vi "AMC Simple Clock Example.vi"() -> ()   [LabVIEW 2017]
uses:
  <vilib>/Utility/config.llb/NI_LVConfig.lvlib
  AMC Simple Clock Style.ctl
  <vilib>/Utility/config.llb/Read Key (I32).vi
  <vilib>/Utility/config.llb/Write Key (I32).vi
panel:
  in  "Save State":bool
  out "Seconds":bool[](array[boolean])
  out "Seconds Tens":bool[](array[boolean])
  out "Minutes":bool[](array[boolean])
  out "Minutes Tens":bool[](array[boolean])
  out "Hours":bool[](array[boolean])
  out "Hours Tens":bool[](array[boolean])
  out "Digital":string
  in  "Clock Style":T1
  out "Hour":dbl(knob) scale=0.0..12.0
  out "Minute":dbl(knob) scale=0.0..12.0 scale format="%#.0f"
  out "Status":string
  in  "About":bool
  in  "Exit":bool
  in  "State Variables":cluster{"Config File":path, "Clock Style":T1}
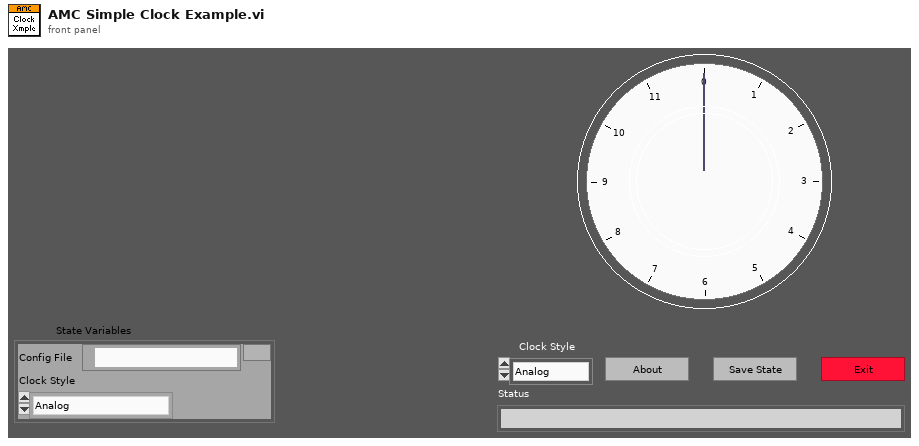
[diagram p1: front panel]
types:
  T1 = typedef "AMC Simple Clock Style.ctl" = enum16{"Analog", "Digital", "Binary"}
  T2 = typedef "amc_Message Queue.ctl" = refnum<queue>
  T3 = typedef "LVDateTimeRec.ctl" = cluster{"fractional second":dbl, "second":i32, "minute":i32, "hour":i32, "day of month":i32, "month":i32, "year":i32, "day of week":i32, "day of year":i32, "DST":i32}
  T4 = typedef "NI_LVConfig.lvlib/Config Data RefNum.ctl" = refnum<k1>
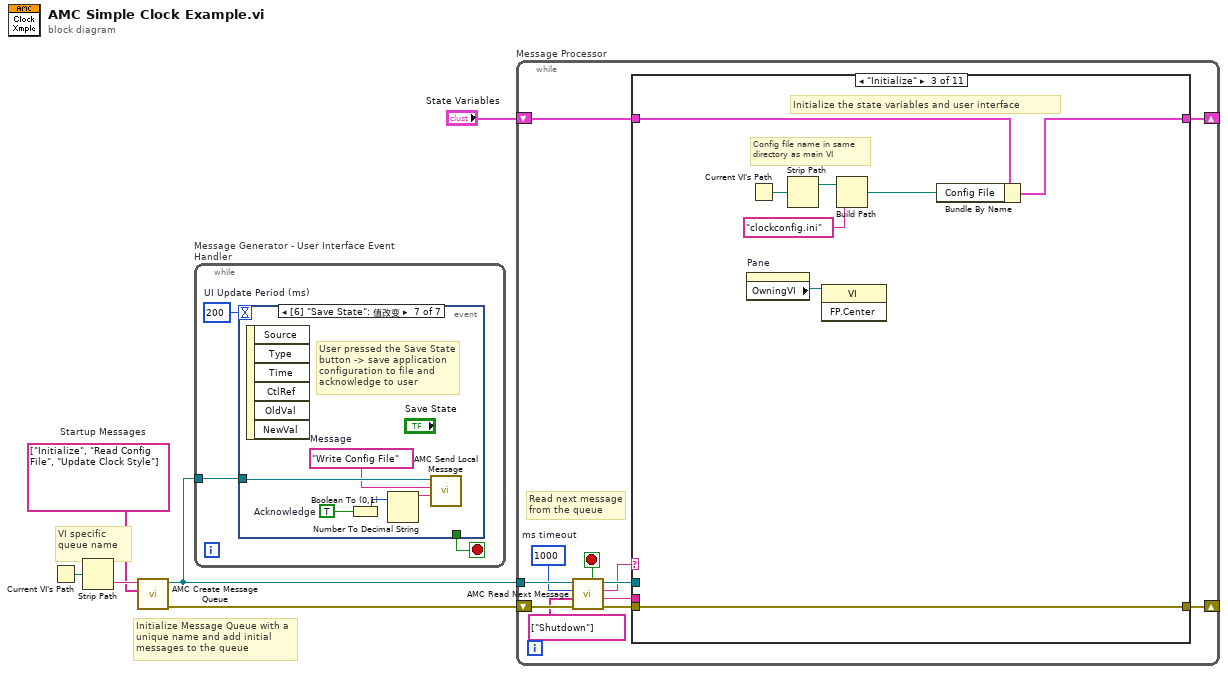
[diagram p0: block diagram]
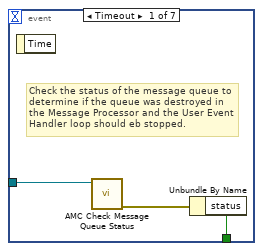
[diagram p2: hidden frame]
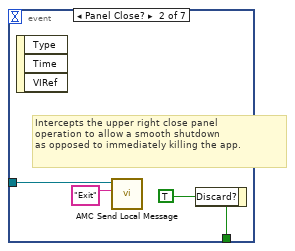
[diagram p3: hidden frame]
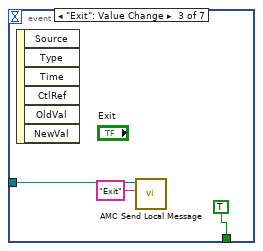
[diagram p4: hidden frame]
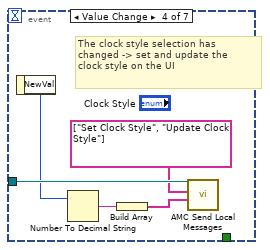
[diagram p5: hidden frame]
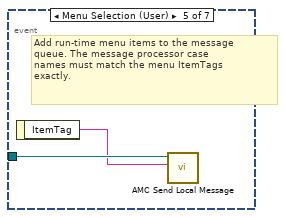
[diagram p6: hidden frame]
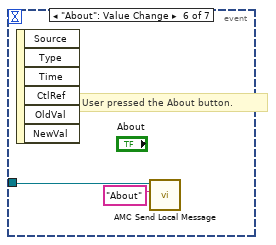
[diagram p7: hidden frame]
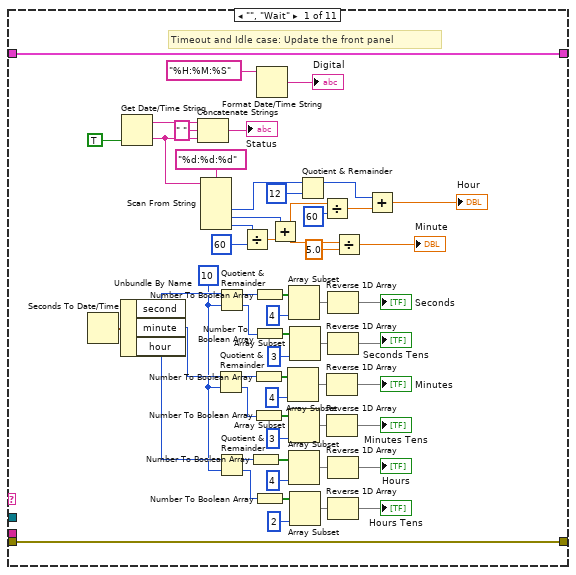
[diagram p8: hidden frame]
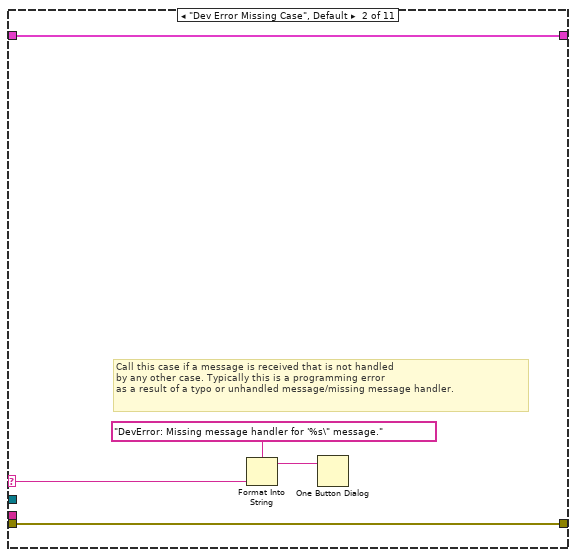
[diagram p9: hidden frame]
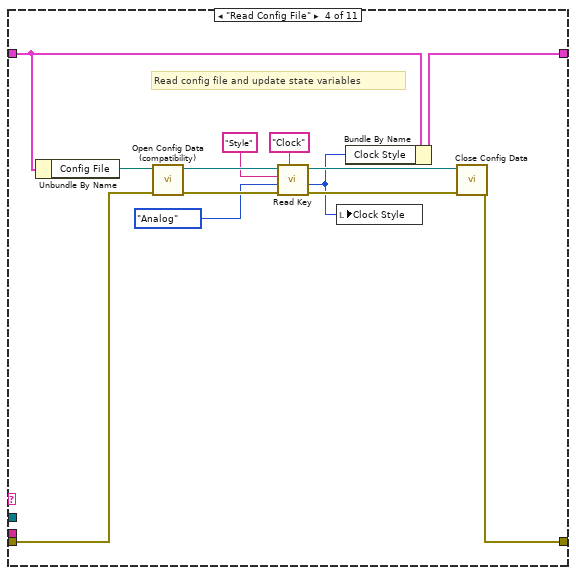
[diagram p10: hidden frame]
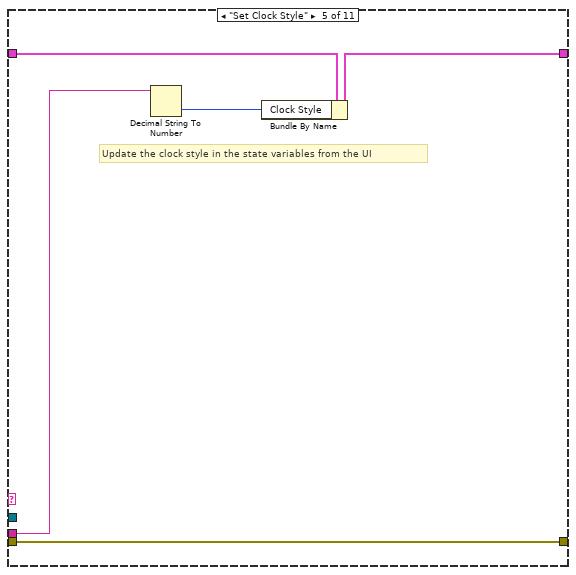
[diagram p11: hidden frame]
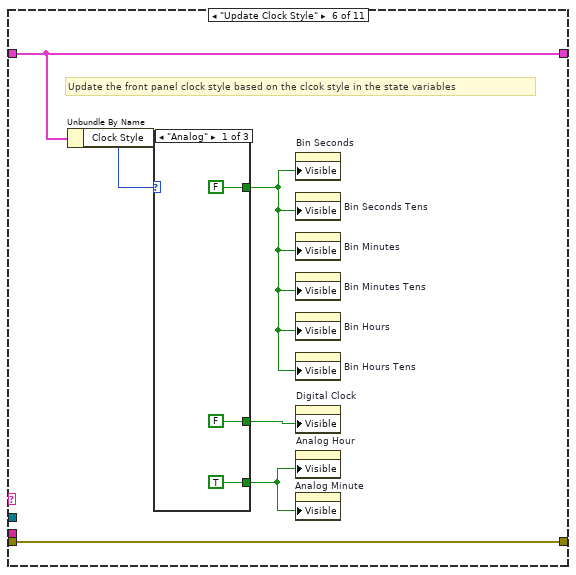
[diagram p12: hidden frame]
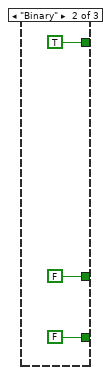
[diagram p13: hidden frame]
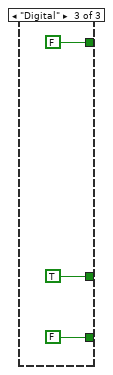
[diagram p14: hidden frame]
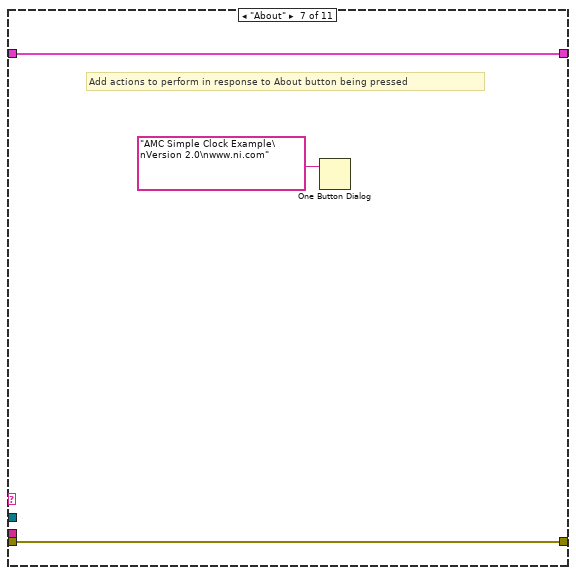
[diagram p15: hidden frame]
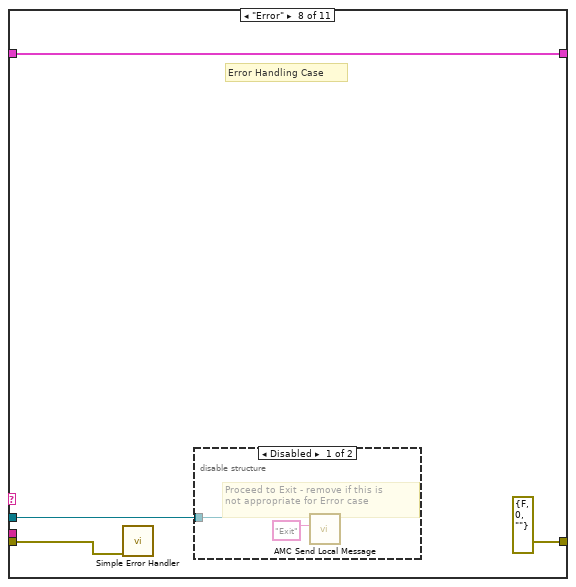
[diagram p16: hidden frame]
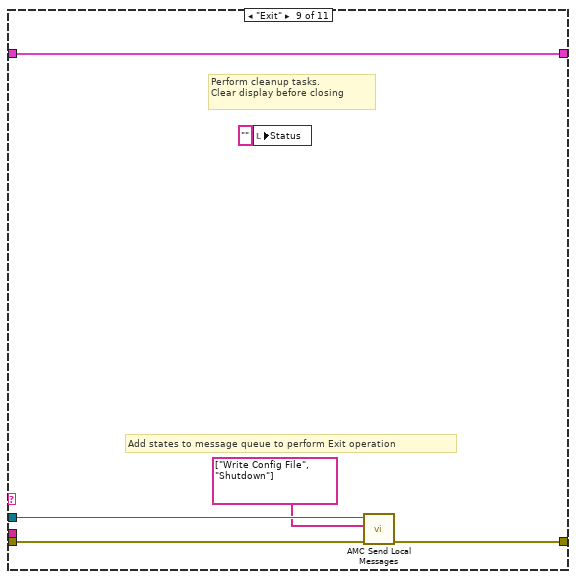
[diagram p18: hidden frame]
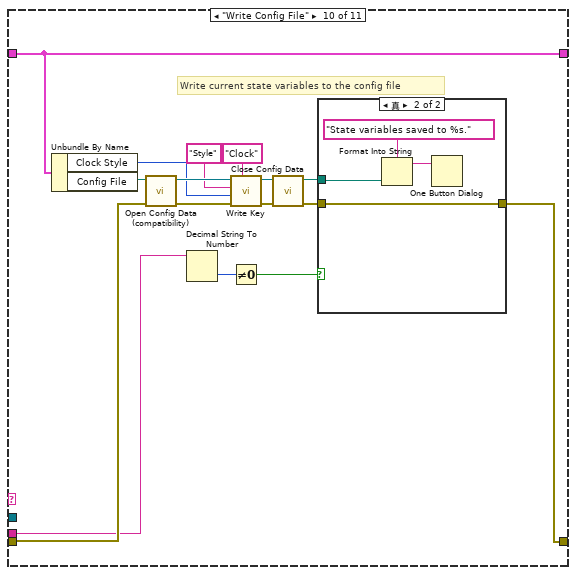
[diagram p19: hidden frame]
diagram:
  w1 = string[] ["Initialize", "Read Config File", "Update Clock Style"]  # Startup Messages
  # "VI specific\nqueue name"
  # "Initialize Message Queue with a unique name and add initial messages to the queue"
  n1 = Current VI's Path() -> (path=w3:path)
  n2 = Strip Path(path=w3) -> (name=w2:string)  [unwired: 1 out]
  n3 = call "AMC Create Message Queue.vi"("Initial Message Names"=w1, "Message Queue Name"=w2) -> ("error out"=w6:errorcluster, "Message Queue out"=w4:T2)  [unwired: 3 in, 5 out]
  n4 = while "Message Generator - User Interface Event Handler" {
    tunnel: w4 -> [w7]
    stop <- w8 stop-if-true
    w9 = 200  # UI Update Period (ms)
    n5 = event shown="[6] \"Save State\": 值改变" {
      selector: _ -> [_ _ _ _ _ _ _]
      dyn-events: _ -> [_ _ _ _ _ _ _]
      timeout: w9 -> [_ _ _ _ _ _ _]
      tunnel: [w12 w15 TRUE ("Discard?") _ _ _ _] -> w8
      tunnel: w7 -> [w11 w14 w17 w23 w25 w27 w32]
      event Timeout {
        # "Check the status of the message queue to determine if the queue was destroyed in the Message Processor and the User Event Handler loop should eb stopped."
        n6 = event-data() -> ()  [unwired: 2 out]
        n7 = call "AMC Check Message Queue Status.vi"("Message queue in"=w11) -> ("error out"=w10:errorcluster)  [unwired: 2 in, 7 out]
        n8 = Unbundle By Name(w10) -> ("status"=w12:bool)
      }
      event Panel Close? {
        w15 = TRUE ("Discard?")
        # "Intercepts the upper right close panel\noperation to allow a smooth shutdown\nas opposed to immediately killing the app."
        n9 = event-data() -> ()  [unwired: 4 out]
        n10 = call "AMC Send Local Message.vi"("Message Name"="Exit", "Message Queue in"=w14) -> ()  [unwired: 4 in, 6 out]
        n11 = event-data("Discard?"=w15) -> ()  [unwired: 1 in, 1 out]
      }
      event "Exit": Value Change {
        n12 = event-data() -> ()  [unwired: 7 out]
        n13 = call "AMC Send Local Message.vi"("Message Name"="Exit", "Message Queue in"=w17) -> ()  [unwired: 4 in, 6 out]
      }
      event Value Change {
        # "The clock style selection has\nchanged -> set and update the\nclock style on the UI"
        n14 = event-data() -> ("NewVal"=w20:T1)  [unwired: 1 out]
        n15 = Number To Decimal String(number=w20) -> (decimal integer string=w22:string)  [unwired: 1 out]
        n16 = Build Array(w22) -> (w21:string[])
        n17 = call "AMC Send Local Messages.vi"("Message Values"=w21, "Message Names"=string[] ["Set Clock Style", "Update Clock Style"], "Message Queue in"=w23) -> ()  [unwired: 2 in, 7 out]
      }
      event Menu Selection (User) {
        # "Add run-time menu items to the message\nqueue. The message processor case\nnames must match the menu ItemTags\nexactly."
        n18 = event-data() -> ("ItemTag"=w24:string)  [unwired: 1 out]
        n19 = call "AMC Send Local Message.vi"("Message Name"=w24, "Message Queue in"=w25) -> ()  [unwired: 4 in, 6 out]
      }
      event "About": Value Change {
        # "User pressed the About button."
        n20 = event-data() -> ()  [unwired: 7 out]
        n21 = call "AMC Send Local Message.vi"("Message Name"="About", "Message Queue in"=w27) -> ()  [unwired: 4 in, 6 out]
      }
      event "Save State": Value Change {
        w30 = TRUE  # Acknowledge
        w31 = "Write Config File"  # Message
        # "User pressed the Save State button -> save application configuration to file and acknowledge to user"
        n22 = event-data() -> ()  [unwired: 7 out]
        n23 = Boolean To (0,1)(Boolean=w30) -> (0, 1=w28:i16)
        n24 = Number To Decimal String(number=w28) -> (decimal integer string=w29:string)  [unwired: 1 out]
        n25 = call "AMC Send Local Message.vi"("Message Value"=w29, "Message Name"=w31, "Message Queue in"=w32) -> ()  [unwired: 3 in, 6 out]
      }
    }
  }
  n26 = while "Message Processor" {
    shift-left: w6 -> [w38]
    shift-right: [w39] -> _
    tunnel: w4 -> [w37]
    shift-left: "State Variables" -> [w44]
    shift-right: [w43] -> _
    stop <- w42 stop-if-true
    w35 = 1000  # ms timeout
    # "Read next message from the queue"
    n27 = call "AMC Read Next Message.vi"("error in (no error)"=w38, "Termination List ([Exit])"=string[] ["Shutdown"], "timeout (1ms)"=w35, "Message Queue in"=w37) -> ("error out"=w40:errorcluster, "Message Value"=w34:string, "Message Name"=w36:string, "Message Queue out"=w41:T2, "Exit Process"=w42:bool)  [unwired: 3 out]
    n28 = case shown="\"Initialize\"" w36 {
      selector: w36 -> [_ w105 _ _ _ _ _ _ _ _ _]
      tunnel: [w102 w107 w113 w124 w131 w138 w150 w155 w163 w171 w186] -> w43
      tunnel: w44 -> [w102 w107 w114 w120 w132 w138 w150 w155 w163 w171 w186]
      tunnel: w41 -> [_ _ _ _ _ _ _ w152 w161 _ w187]
      tunnel: w40 -> [w101 w106 w115 w118 w133 w139 w151 w153 w160 w170 w188]
      tunnel: [w101 w106 w115 w117 w133 w139 w151 errorcluster {"status"=FALSE, "code"=0, "source"=""} ("error out") w159 w164 w185] -> w39
      tunnel: w34 -> [_ _ _ _ w130 _ _ _ _ w169 _]
      frame "", "Wait" {
        w59 = 10 ("y")
        # "Timeout and Idle case: Update the front panel"
        n29 = Seconds To Date/Time() -> (date time rec=w85:T3)  [unwired: 2 out]
        n30 = Unbundle By Name(w85) -> ("second"=w84:i32, "minute"=w61:i32, "hour"=w60:i32)
        n31 = Get Date/Time String(want seconds? (F)=TRUE) -> (date string=w100:string, time string=w50:string)  [unwired: 2 out]
        n32 = Concatenate Strings(w100, " " ("string"), w50) -> (→"Status":string)
        n33 = Scan From String(format string="%d:%d:%d", input string=w50) -> (output 1=w46:i32, output 2=w93:i32, output 3=w86:i32)  [unwired: 2 in, 6 out]
        n34 = Quotient & Remainder(x=w61, y=w59) -> (x-y*floor(x/y)=w52:i32, floor(x/y)=w68:i32)
        n35 = Quotient & Remainder(x=w84, y=w59) -> (x-y*floor(x/y)=w83:i32, floor(x/y)=w82:i32)
        n36 = Quotient & Remainder(x=w60, y=w59) -> (x-y*floor(x/y)=w57:i32, floor(x/y)=w67:i32)
        n37 = Divide(x=w86, y=60) -> (x/y=w94:dbl)
        n38 = Number To Boolean Array(number=w57) -> (Boolean array=w56:bool[])
        n39 = Number To Boolean Array(number=w52) -> (Boolean array=w51:bool[])
        n40 = Number To Boolean Array(number=w68) -> (Boolean array=w72:bool[])
        n41 = Number To Boolean Array(number=w83) -> (Boolean array=w80:bool[])
        n42 = Number To Boolean Array(number=w82) -> (Boolean array=w77:bool[])
        n43 = Number To Boolean Array(number=w67) -> (Boolean array=w63:bool[])
        n44 = Format Date/Time String(time format string (%c)="%H:%M:%S") -> (date/time string=→"Digital":string)  [unwired: 2 out]
        n45 = Add(x=w93, y=w94) -> (x+y=w89:dbl)
        n46 = Array Subset(array=w51, length=4) -> (w69:bool[])  [unwired: 1 in]
        n47 = Array Subset(array=w80, length=4) -> (w81:bool[])  [unwired: 1 in]
        n48 = Array Subset(array=w72, length=3) -> (w73:bool[])  [unwired: 1 in]
        n49 = Array Subset(array=w56, length=4) -> (w66:bool[])  [unwired: 1 in]
        n50 = Array Subset(array=w77, length=3) -> (w76:bool[])  [unwired: 1 in]
        n51 = Array Subset(array=w63, length=2) -> (w62:bool[])  [unwired: 1 in]
        n52 = Quotient & Remainder(x=w46, y=12) -> (x-y*floor(x/y)=w45:i32)  [unwired: 1 out]
        n53 = Divide(x=w89, y=60) -> (x/y=w91:dbl)
        n54 = Reverse 1D Array(array=w69) -> (reversed array=→"Minutes":bool[])
        n55 = Reverse 1D Array(array=w73) -> (reversed array=→"Minutes Tens":bool[])
        n56 = Reverse 1D Array(array=w81) -> (reversed array=→"Seconds":bool[])
        n57 = Reverse 1D Array(array=w76) -> (reversed array=→"Seconds Tens":bool[])
        n58 = Reverse 1D Array(array=w66) -> (reversed array=→"Hours":bool[])
        n59 = Reverse 1D Array(array=w62) -> (reversed array=→"Hours Tens":bool[])
        n60 = Divide(x=w89, y=5.0) -> (x/y=→"Minute":dbl)
        n61 = Add(x=w45, y=w91) -> (x+y=→"Hour":dbl)
      }
      frame "Dev Error Missing Case", Default {
        # "Call this case if a message is received that is not handled \nby any other case. Typically this is a programming error\nas a result of a typo or unhandled message/missing message handler."
        n62 = Format Into String(format string="DevError: Missing message handler for '%s\" message." ("message"), w105) -> (resulting string=w103:string)  [unwired: 2 in, 1 out]
        n63 = One Button Dialog(message=w103) -> ()  [unwired: 2 out]
      }
      frame "Initialize" {
        # "Config file name in same directory as main VI"
        # "Initialize the state variables and user interface"
        n64 = property on="Pane" class="Pane"() -> ("OwningVI"=w108:refnum<vi>)  [unwired: 2 in, 2 out]
        n65 = Current VI's Path() -> (path=w112:path)
        n66 = Strip Path(path=w112) -> (stripped path=w111:path)  [unwired: 1 out]
        n67 = invoke class="VI" method="FP.Center"(reference=w108) -> ()  [unwired: 2 in, 3 out]
        n68 = Build Path(base path=w111, name or relative path="clockconfig.ini") -> (appended path=w109:path)
        n69 = Bundle By Name(cluster=w114, "Config File"=w109) -> (w113:cluster{"Config File":path, "Clock Style":T1})
      }
      frame "Read Config File" {
        # "Read config file and update state variables"
        n70 = Unbundle By Name(w120) -> ("Config File"=w119:path)
        n71 = call <vilib>:"Open Config Data (compatibility).vi"("error in (no error)"=w118, "configuration file path"=w119) -> ("error out"=w128:errorcluster, "refnum"=w127:T4)  [unwired: 7 in, 1 out]
        n72 = call-poly <vilib>:"Read Key.vi"("section"="Clock", "error in (no error)"=w128, "default value"=AMC_Simple_Clock_Style."Analog" ("NewVal"), "key"="Style", "refnum"=w127) -> ("error out"=w121:errorcluster, "value"=w116:i32, "refnum out"=w122:T4)  [unwired: 4 out]
        n73 = local write "Clock Style"(w116) -> ()
        n74 = Bundle By Name(cluster=w120, "Clock Style"=w116) -> (w124:cluster{"Config File":path, "Clock Style":T1})
        n75 = call <vilib>:"Close Config Data.vi"("error in (no error)"=w121, "refnum"=w122) -> ("error out"=w117:errorcluster)  [unwired: 1 in, 8 out]
      }
      frame "Set Clock Style" {
        # "Update the clock style in the state variables from the UI"
        n76 = Decimal String To Number(string=w130) -> (number=w129:i32)  [unwired: 3 out]
        n77 = Bundle By Name(cluster=w132, "Clock Style"=w129) -> (w131:cluster{"Config File":path, "Clock Style":T1})
      }
      frame "Update Clock Style" {
        # "Update the front panel clock style based on the clcok style in the state variables"
        n78 = Unbundle By Name(w138) -> ("Clock Style"=w137:T1)
        n79 = case shown="\"Analog\"" w137 {
          tunnel: [FALSE FALSE TRUE] -> w136
          tunnel: [TRUE FALSE FALSE] -> w135
          tunnel: [FALSE TRUE FALSE] -> w134
          frame "Analog" {
          }
          frame "Binary" {
          }
          frame "Digital" {
          }
        }
        n80 = property on="Bin Seconds" class="Arr (严格)"("Visible"=w134) -> ()  [unwired: 2 in, 2 out]
        n81 = property on="Bin Seconds Tens" class="Arr (严格)"("Visible"=w134) -> ()  [unwired: 2 in, 2 out]
        n82 = property on="Bin Minutes" class="Arr (严格)"("Visible"=w134) -> ()  [unwired: 2 in, 2 out]
        n83 = property on="Bin Minutes Tens" class="Arr (严格)"("Visible"=w134) -> ()  [unwired: 2 in, 2 out]
        n84 = property on="Bin Hours" class="Arr (严格)"("Visible"=w134) -> ()  [unwired: 2 in, 2 out]
        n85 = property on="Bin Hours Tens" class="Arr (严格)"("Visible"=w134) -> ()  [unwired: 2 in, 2 out]
        n86 = property on="Digital Clock" class="Str"("Visible"=w136) -> ()  [unwired: 2 in, 2 out]
        n87 = property on="Analog Hour" class="Knob (严格)"("Visible"=w135) -> ()  [unwired: 2 in, 2 out]
        n88 = property on="Analog Minute" class="Knob (严格)"("Visible"=w135) -> ()  [unwired: 2 in, 2 out]
      }
      frame "About" {
        # "Add actions to perform in response to About button being pressed"
        n89 = One Button Dialog(message="AMC Simple Clock Example\nVersion 2.0\nwww.ni.com") -> ()  [unwired: 2 out]
      }
      frame "Error" {
        # "Error Handling Case"
        n90 = call <vilib>:"Simple Error Handler.vi"("error in (no error)"=w153) -> ()  [unwired: 1 in, 8 out]
        n91 = disable-structure shown="Disabled" {
          disable-tunnel: w152 -> [w157 _]
          frame Disabled {
            # "Proceed to Exit - remove if this is\nnot appropriate for Error case"
            n92 = call "AMC Send Local Message.vi"("Message Name"="Exit", "Message Queue in"=w157) -> ()  [unwired: 8 in, 2 out]
          }
          frame Enabled {
          }
        }
      }
      frame "Exit" {
        # "Add states to message queue to perform Exit operation"
        # "Perform cleanup tasks.\nClear display before closing"
        n93 = local write "Status"("" ("Status")) -> ()
        n94 = call "AMC Send Local Messages.vi"("error in (no error)"=w160, "Message Names"=string[] ["Write Config File", "Shutdown"], "Message Queue in"=w161) -> ("error out"=w159:errorcluster)  [unwired: 2 in, 6 out]
      }
      frame "Write Config File" {
        # "Write current state variables to the config file"
        n95 = Unbundle By Name(w171) -> ("Clock Style"=w172:T1, "Config File"=w173:path)
        n96 = call <vilib>:"Open Config Data (compatibility).vi"("error in (no error)"=w170, "configuration file path"=w173) -> ("error out"=w179:errorcluster, "refnum"=w178:T4)  [unwired: 7 in, 1 out]
        n97 = Decimal String To Number(string=w169) -> (number=w168:i32)  [unwired: 3 out]
        n98 = call-poly <vilib>:"Write Key.vi"("section"="Clock", "error in (no error)"=w179, "value"=w172, "key"="Style", "refnum"=w178) -> ("error out"=w174:errorcluster, "refnum out"=w175:T4)  [unwired: 5 out]
        n99 = Not Equal To 0?(x=w168) -> (x != 0?=w167:bool)
        n100 = call <vilib>:"Close Config Data.vi"("error in (no error)"=w174, "refnum"=w175) -> ("error out"=w166:errorcluster, "file path"=w165:path)  [unwired: 1 in, 7 out]
        n101 = case shown="真" w167 {
          tunnel: w166 -> [w180 w181]
          tunnel: w165 -> [_ w184]
          tunnel: [w180 w181] -> w164
          frame False {
          }
          frame True {
            n102 = Format Into String(format string="State variables saved to %s.", w184) -> (resulting string=w182:string)  [unwired: 2 in, 1 out]
            n103 = One Button Dialog(message=w182) -> ()  [unwired: 2 out]
          }
        }
      }
      frame "Shutdown" {
        n104 = call "AMC Destroy Message Queue.vi"("error in (no error)"=w188, "Message Queue in"=w187) -> ("error out"=w185:errorcluster)  [unwired: 9 out]
      }
    }
  }
